vi "FileLoad.vi"   [LabVIEW 2014]
uses:
  commandCluster.ctl
  Robot Global Data.vi
types:
  T1 = typedef "commandCluster.ctl" = cluster{"Step ID":i32, "Command Type":i32, "Drive X":dbl, "Drive Y":dbl, "Heading":dbl, "Max Exec. Time":dbl, "Jump Type":i32, "Jump To":i32, "Jump Condition":i32}
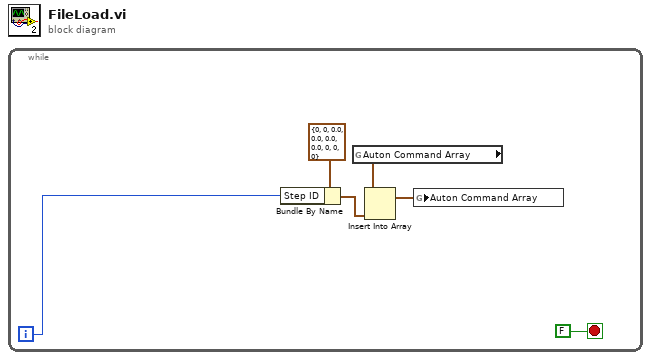
[diagram p0: block diagram]
diagram:
  n1 = while {
    i -> [w2]
    stop <- FALSE stop-if-true
    n2 = Bundle By Name(cluster=T1 {"Step ID"=0, "Command Type"=0, "Drive X"=0.0, "Drive Y"=0.0, "Heading"=0.0, "Max Exec. Time"=0.0, "Jump Type"=0, "Jump To"=0, "Jump Condition"=0} ("Command Cluster"), "Step ID"=w2) -> (w4:T1)
    n3 = global read "Robot Global Data.vi" "Auton Command Array"() -> (w5:T1[])
    n4 = Insert Into Array(array=w5, new element=w4) -> (w6:T1[])  [unwired: 1 in]
    n5 = global write "Robot Global Data.vi" "Auton Command Array"(w6) -> ()
  }
